vi "Compare.vi"(8 "error in":errorcluster, 10 "Actual":refnum<class "CANopen Response Message.lvclass">, 11 "Upload Segment Response Comparator in":refnum<class "Upload Segment Response Comparator.lvclass">) -> (0 "error out":errorcluster, 2 "Equal?":bool, 3 "Upload Segment Response Comparator out":refnum<class "Upload Segment Response Comparator.lvclass">)   [LabVIEW 2024, in "CANopen Master.lvlib" / "Upload Segment Response Comparator.lvclass"]
uses:
  Upload Segment Response Comparator.lvclass
  Upload Segment Response Comparator.lvclass/Upload Segment Response Comparator.ctl
  SDO Response Compare Strategy/SDO Response Compare Strategy.lvclass
  CANopen Response/CANopen Response Message.lvclass
  D:/git/CANopen-XNET/SDO Response Compare Strategy/SDO Response Compare Strategy.lvclass
  D:/git/CANopen-XNET/Upload Segment Response Comparator/Upload Segment Response Comparator.lvclass
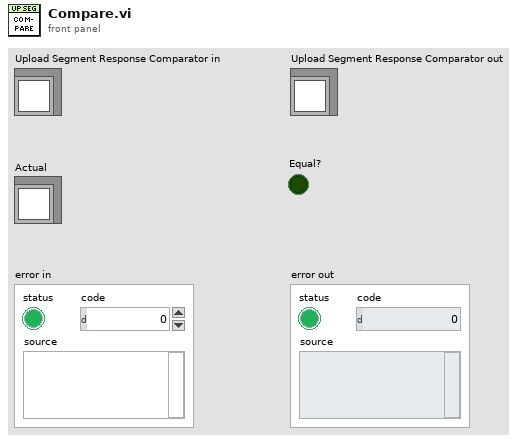
[diagram p1: front panel]
types:
  T1 = typedef "CANopen Master.lvlib/CANopen Response Message.lvclass/Server Command Specifier.ctl" = enum8{"Upload Segment Response", "Download Segment Response", "Initiate Upload Response", "Initiate Download Response", "Heartbeat", "Block Download"}
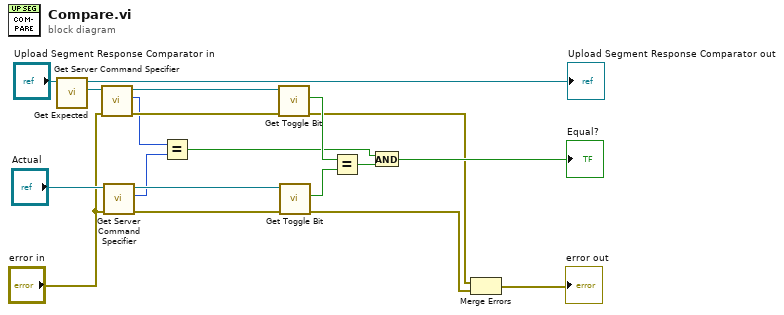
[diagram p0: block diagram]
diagram:
  n1 = call "Get Expected.vi"("SDO Response Compare Strategy in"="Upload Segment Response Comparator in") -> ("Expected Response Message"=w16:refnum<class "CANopen Response Message.lvclass">, "SDO Response Compare Strategy out"=→"Upload Segment Response Comparator out":refnum<class "Upload Segment Response Comparator.lvclass">)  [unwired: 9 in]
  n2 = call-dynamic "Get Server Command Specifier.vi"("error in"="error in", "CANopen Response in"=w16) -> ("error out"=w11:errorcluster, "Server Command Specifier"=w9:T1, "CANopen Response out"=w13:refnum<class "CANopen Response Message.lvclass">)  [unwired: 7 in]
  n3 = call-dynamic "Get Server Command Specifier.vi"("error in"="error in", "CANopen Response in"="Actual") -> ("error out"=w4:errorcluster, "Server Command Specifier"=w8:T1, "CANopen Response out"=w12:refnum<class "CANopen Response Message.lvclass">)  [unwired: 7 in]
  n4 = Equal?(x=w9, y=w8) -> (x = y?=w6:bool)
  n5 = call-dynamic "Get Toggle Bit.vi"("error in"=w11, "CANopen Response Message in"=w13) -> ("error out"=w2:errorcluster, "Toggle-Bit"=w15:bool)  [unwired: 7 in, 1 out]
  n6 = call-dynamic "Get Toggle Bit.vi"("error in"=w4, "CANopen Response Message in"=w12) -> ("error out"=w3:errorcluster, "Toggle-Bit"=w14:bool)  [unwired: 7 in, 1 out]
  n7 = Equal?(x=w15, y=w14) -> (x = y?=w7:bool)
  n8 = And(x=w6, y=w7) -> (x .and. y?=→"Equal?":bool)
  n9 = Merge Errors(w2, w3) -> (→"error out":errorcluster)
